vi "fxp_to_fp.vi"() -> ()   [LabVIEW 2018]
uses:
  <vilib>/Platform/TimedLoop/XDataNode/timing_clust.ctl
  <vilib>/Platform/TimedLoop/XDataNode/nitl_modes.ctl
  <vilib>/Platform/TimedLoop/XDataNode/wakeup.ctl
  <vilib>/rvi/Emulation/niFpgaGetClockAttributes.vi
  <vilib>/rvi/Emulation/niFpgaSctlEmulationGetInTimedLoop.vi
  <vilib>/rvi/Emulation/niFpgaEmulationReportErrorSimple.vi
  <vilib>/rvi/Emulation/niFpgaProcessEmulError.vi
  <vilib>/rvi/Emulation/niFpgaCriticalErrorInLSC.vi
  <vilib>/Platform/TimedLoop/XDataNode/XDataNode.xnode
  <vilib>/Platform/TimedLoop/XDataNode/XDNodeRunTimeDep.lvlib
panel:
  out "single precision float 7":sgl
  out "single precision float 6":sgl
  out "single precision float 5":sgl
  out "single precision float 4":sgl
  out "single precision float 3":sgl
  out "single precision float 2":sgl
  out "single precision float":sgl
  in  "stop 2":bool
  in  "stop":bool
  out "Numeric 16":fxp<+/-,16,16>
  in  "Numeric 15":fxp<+/-,16,16>
  out "Numeric 14":fxp<+/-,16,16>
  in  "Numeric 13":fxp<+/-,16,16>
  out "Numeric 12":fxp<+/-,16,16>
  in  "Numeric 11":fxp<+/-,16,16>
  out "Numeric 10":fxp<+/-,16,16>
  in  "Numeric 9":fxp<+/-,16,16>
  out "Numeric 8":fxp<+/-,16,16>
  in  "Numeric 7":fxp<+/-,16,16>
  out "Numeric 6":fxp<+/-,16,16>
  in  "Numeric 5":fxp<+/-,16,16>
  out "Numeric 4":fxp<+/-,16,16>
  in  "Numeric 3":fxp<+/-,16,16>
  out "Numeric 2":fxp<+/-,16,16>
  in  "Numeric":fxp<+/-,16,16>
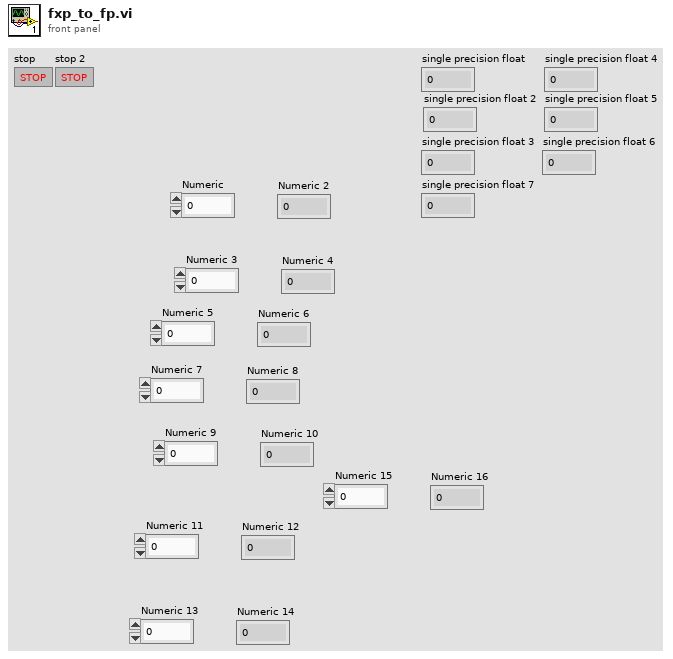
[diagram p1: front panel]
types:
  T1 = typedef "XDNodeRunTimeDep.lvlib/timing_clust.ctl" = cluster{"Expected End [f-1]":u64, "Actual End [f-1]":u64, "Finished Late? [f-1]":bool, "Expected End [i-1]":u64, "Actual End [i-1]":u64, "Finished Late? [i-1]":bool, "Expected Start [i]":u64, "Actual Start [i]":u64, "Expected Start [f]":u64, "Actual Start [f]":u64, "Source Name":string, "Structure Name":string, "Period":i64, "Deadline":i64, "Offset":i64, "Start":i64, "Priority":i32, "Timeout":i32, "Mode":T2, "Wakeup Reason":T3, "Error":errorcluster, "Source Type":string, "Secondary Source Type":string, "Global End Time":u64, "Global Start Time":u64, "Frame Duration":u64, "Iteration Duration":u64, "Assigned CPU":i32, "I/O Scan Engine Mode":u32}
  T2 = typedef "XDNodeRunTimeDep.lvlib/nitl_modes.ctl" = enum32{"No Change", "Process missed periods, maintain original phase", "Discard missed periods, maintain original phase", "Process missed periods, ignore original phase", "Discard missed periods, ignore original phase"}
  T3 = typedef "XDNodeRunTimeDep.lvlib/wakeup.ctl" = enum32{"Normal", "Aborted", "Asynchronous wakeup", "Timing source error", "Timed loop error", "Timeout"}
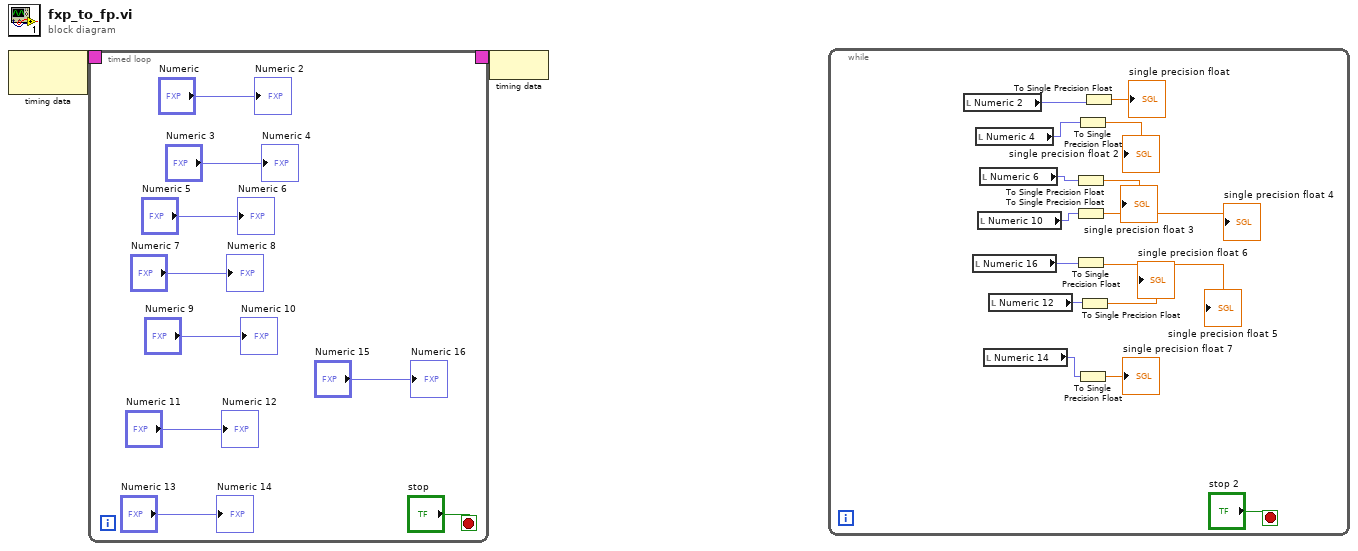
[diagram p0: block diagram]
diagram:
  n1 = node-c288() -> (w2:T1)  [unwired: 1 in]
  n2 = timed-loop {
    timing: w2 -> [_]
    timing-out: [_] -> w1
    stop <- "stop" stop-if-true
    "Numeric 2" <- "Numeric"
    "Numeric 4" <- "Numeric 3"
    "Numeric 6" <- "Numeric 5"
    "Numeric 8" <- "Numeric 7"
    "Numeric 10" <- "Numeric 9"
    "Numeric 12" <- "Numeric 11"
    "Numeric 14" <- "Numeric 13"
    "Numeric 16" <- "Numeric 15"
  }
  n3 = node-c288(w1) -> ()
  n4 = while {
    stop <- "stop 2" stop-if-true
    n5 = local read "Numeric 2"() -> (w27:fxp<+/-,16,16>)
    n6 = local read "Numeric 16"() -> (w23:fxp<+/-,16,16>)
    n7 = local read "Numeric 4"() -> (w26:fxp<+/-,16,16>)
    n8 = local read "Numeric 10"() -> (w24:fxp<+/-,16,16>)
    n9 = local read "Numeric 6"() -> (w25:fxp<+/-,16,16>)
    n10 = local read "Numeric 14"() -> (w21:fxp<+/-,16,16>)
    n11 = local read "Numeric 12"() -> (w22:fxp<+/-,16,16>)
    n12 = To Single Precision Float(number=w25) -> (single precision float=→"single precision float 3":sgl)
    n13 = To Single Precision Float(number=w24) -> (single precision float=→"single precision float 4":sgl)
    n14 = To Single Precision Float(number=w23) -> (single precision float=→"single precision float 5":sgl)
    n15 = To Single Precision Float(number=w26) -> (single precision float=→"single precision float 2":sgl)
    n16 = To Single Precision Float(number=w21) -> (single precision float=→"single precision float 7":sgl)
    n17 = To Single Precision Float(number=w22) -> (single precision float=→"single precision float 6":sgl)
    n18 = To Single Precision Float(number=w27) -> (single precision float=→"single precision float":sgl)
  }
